vi "FGEN Configure Channel.vi"(8 "error in (no error)":errorcluster, 10 "Active Channel":string, 11 "Function Generator in":refnum<class "Function Generator.lvclass">) -> (0 "error out":errorcluster, 3 "Function Generator out":refnum<class "Function Generator.lvclass">)   [LabVIEW 2023, in "HardwareAbstractionLayer_LVOOP.lvlib" / "Function Generator.lvclass"]
uses:
  Function Generator.lvclass
  Function Generator.lvclass/Function Generator.ctl
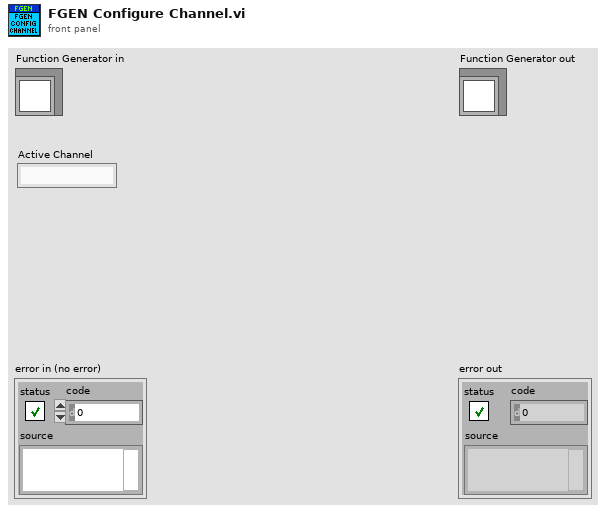
[diagram p1: front panel]
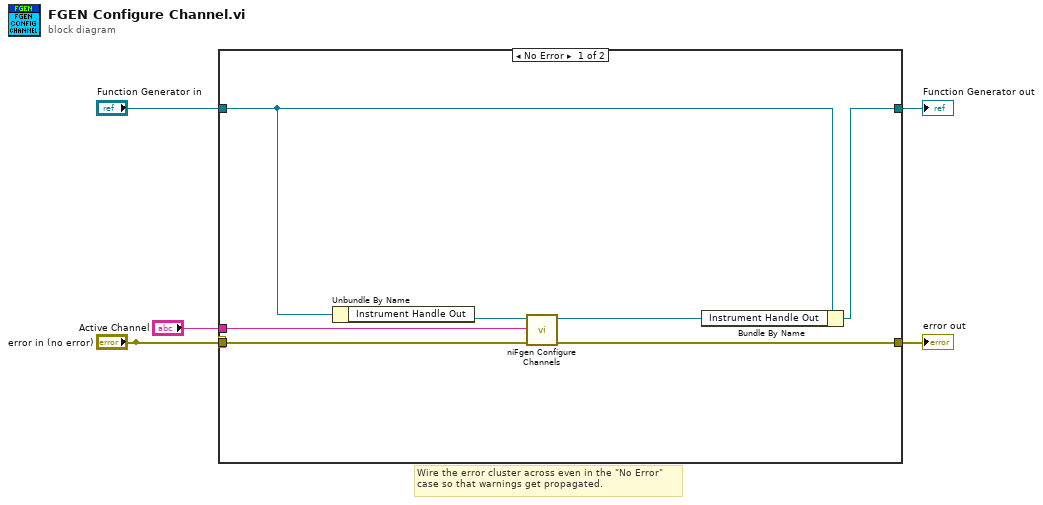
[diagram p0: block diagram]
diagram:
  # "Wire the error cluster across even in the \"No Error\"\ncase so that warnings get propagated."
  n1 = case shown="No Error" "error in (no error)" {
    selector: "error in (no error)" -> [w7 w14]
    tunnel: [w8 w14] -> w5
    tunnel: [w11 w13] -> w3
    tunnel: "Function Generator in" -> [w12 w13]
    tunnel: "Active Channel" -> [w6 _]
    tunnel: "error in (no error)" -> [_ _]
    frame No Error {
      n2 = Unbundle By Name(w12) -> ("Instrument Handle Out"=w10:refnum<k15>)
      n3 = call <instrlib>:"niFgen Configure Channels.vi"("error in (no error)"=w7, "Channels"=w6, "Instrument Handle"=w10) -> ("error out"=w8:errorcluster, "Instrument Handle Out"=w9:refnum<k15>)  [unwired: 7 in]
      n4 = Bundle By Name(cluster=w12, "Instrument Handle Out"=w9) -> (w11:refnum<class "Function Generator.lvclass">)
    }
    frame Error {
    }
  }
  "error out" <- w5
  "Function Generator out" <- w3
